vi "Command Type.vi"(11 "Stop Log Command Config in":refnum<class "Stop Log Command Config.lvclass">) -> (2 "Command Type":string)   [LabVIEW 2020, in "VolatusSeqConfig.lvlib" / "Stop Log Command Config.lvclass"]
uses:
  Stop Log Command Config.lvclass
  Stop Log Command Config.lvclass/Stop Log Command Config.ctl
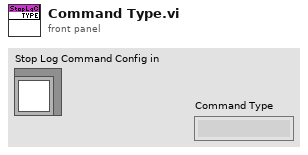
[diagram p1: front panel]
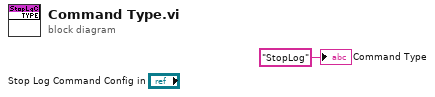
[diagram p0: block diagram]
diagram:
  "Command Type" <- "StopLog" ("Command Type")
